vi "PseudoInverse Calculator.vi"(8 "R4":dbl[](array[numeric]), 9 "R3":dbl[](array[numeric]), 10 "R2":dbl[](array[numeric]), 11 "R1":dbl[](array[numeric])) -> (3 "Pseudoinverse":T1)   [LabVIEW 2020]
uses:
  <vilib>/Analysis/Matrix/Datatypes/RealMatrix.ctl
  <vilib>/Analysis/_algsub.llb/Real PseudoInverse Matrix.vi
  <vilib>/Analysis/NI_AALPro.lvlib
  <vilib>/Analysis/Matrix/NI_Matrix.lvlib
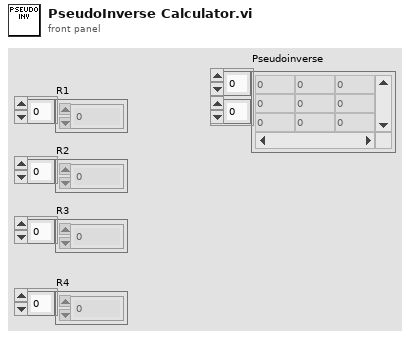
[diagram p1: front panel]
types:
  T1 = typedef "NI_Matrix.lvlib/RealMatrix.ctl" = dbl[][]
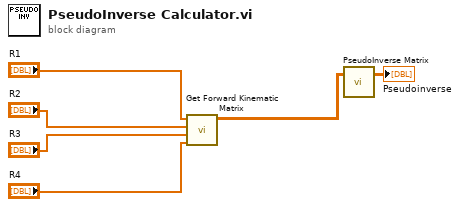
[diagram p0: block diagram]
diagram:
  n1 = call "Get Forward Kinematic Matrix.vi"("R4"="R4", "R3"="R3", "R2"="R2", "R1"="R1") -> ("Real Matrix"=w3:T1)  [unwired: 7 in]
  n2 = call-poly <vilib>:"PseudoInverse Matrix.vi"("Input Matrix"=w3) -> ("PseudoInverse Matrix"=→"Pseudoinverse":T1)  [unwired: 1 in, 1 out]
